vi "ddeserverecive.vi"() -> ()   [LabVIEW 2018]
panel:
  out "topic 2":string="labdata"
  out "service 2":string="labview"
  out "item":string="lovely"
  out "value":string
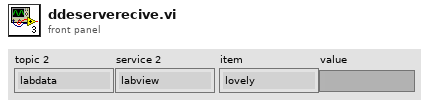
[diagram p1: front panel]
types:
  T1 = enum16{"open", "replace", "create", "open or create", "replace or create", "replace or create with confirmation"}
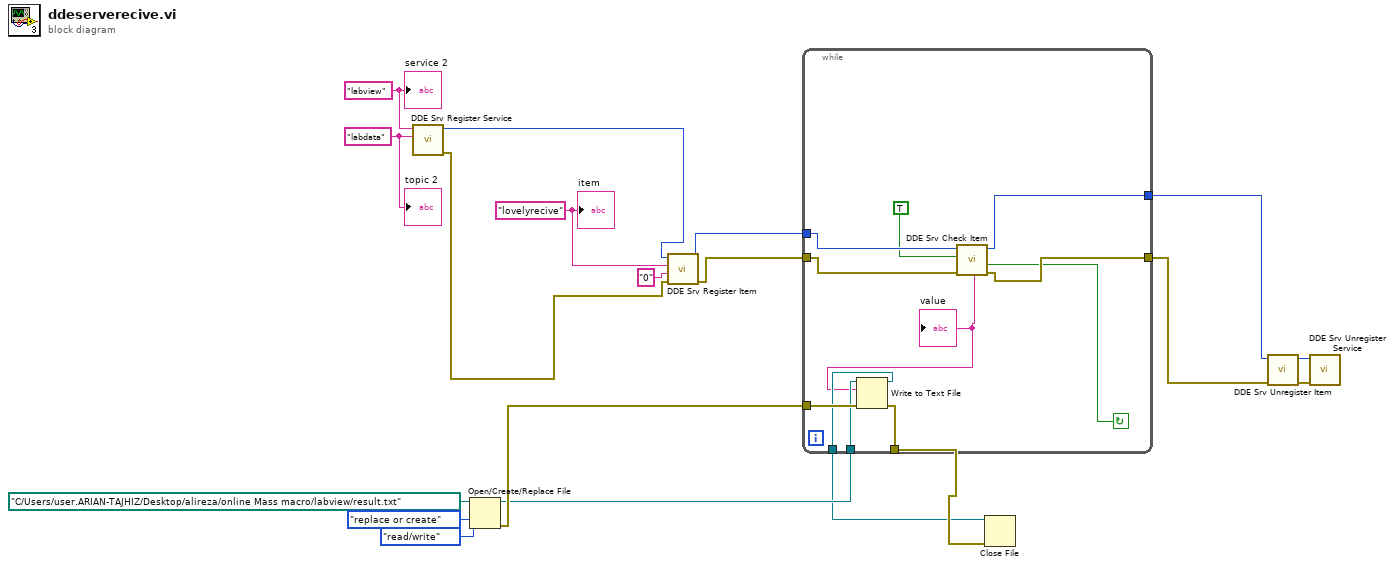
[diagram p0: block diagram]
diagram:
  w10 = "labdata" ("topic")
  w11 = "labview" ("service")
  w13 = "lovelyrecive" ("item")
  n1 = call <vilib>:"DDE Srv Register Service.vi"("topic"=w10, "service"=w11) -> ("error out"=w8:errorcluster, "service refnum"=w9:u32)  [unwired: 6 in]
  n2 = Open/Create/Replace File(file path (use dialog)=path "C:/Users/user.ARIAN-TAJHIZ/Desktop/alireza/online Mass macro/labview/result.txt", operation (0:open)=T1."replace or create", access (0:read/write)=enum16{"read/write", "read-only", "write-only"}."read/write") -> (refnum out=w3:refnum<file>, error out=w4:errorcluster)  [unwired: 3 in, 1 out]
  n3 = call <vilib>:"DDE Srv Register Item.vi"("error in (no error)"=w8, "value"="0", "item"=w13, "service refnum"=w9) -> ("error out"=w14:errorcluster, "item refnum"=w19:u32)  [unwired: 4 in]
  n4 = while {
    tunnel: w19 -> [w30]
    tunnel: [w29] -> w18
    tunnel: w14 -> [w27]
    tunnel: [w28] -> w15
    tunnel: w4 -> [w24]
    tunnel: w3 -> [w23]
    tunnel: [w22] -> w2
    tunnel: [w21] -> w1
    stop <- w25 continue-if-true
    n5 = call <vilib>:"DDE Srv Check Item.vi"("error in (no error)"=w27, "wait for poke(FALSE)"=TRUE, "item refnum in"=w30) -> ("error out"=w28:errorcluster, "poked?"=w25:bool, "value"=w20:string, "item refnum out"=w29:u32)  [unwired: 3 in]
    "value" <- w20
    n6 = Write to Text File(file (use dialog)=w23, text=w20, error in=w24) -> (refnum out=w21:refnum<file>, error out=w22:errorcluster)  [unwired: 1 in, 1 out]
  }
  n7 = Close File(refnum=w1, error in=w2) -> ()  [unwired: 2 out]
  n8 = call <vilib>:"DDE Srv Unregister Item.vi"("error in (no error)"=w15, "item refnum"=w18) -> ("error out"=w16:errorcluster, "service refnum"=w17:u32)  [unwired: 6 in]
  n9 = call <vilib>:"DDE Srv Unregister Service.vi"("error in (no error)"=w16, "service refnum"=w17) -> ()  [unwired: 7 in, 1 out]
  "item" <- w13
  "service 2" <- w11
  "topic 2" <- w10
